vi "Euler Project Problem 3 Solution.vi"() -> ()   [LabVIEW 2011]
uses:
  <vilib>/gmath/NI_AAL_MathFunc.lvlib
panel:
  out "Max prime value":i64
  in  "n":i64=600851475143
  # "Problem Description:\n\nFind the largest palindrome made from the product of two 3-digit numbers."
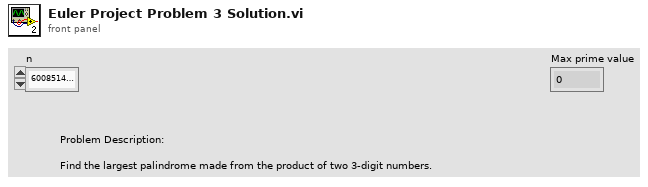
[diagram p1: front panel]
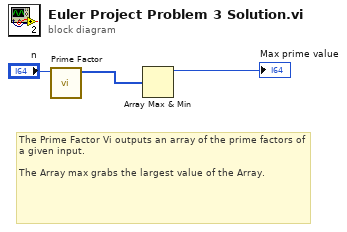
[diagram p0: block diagram]
diagram:
  # "The Prime Factor Vi outputs an array of the prime factors of a given input. \n\nThe Array max grabs the largest value of the Array."
  n1 = call <vilib>:"Prime Factor.vi"("n"="n") -> ("Prime Factors"=w2:i64[])  [unwired: 9 in]
  n2 = Array Max & Min(array=w2) -> (max value=→"Max prime value":i64)  [unwired: 3 out]
